vi "Blob ReadEdvr.vi"(8 "error in (no error)":errorcluster, 11 "Blob in":refnum<class "Blob.lvclass">) -> (0 "error out":errorcluster, 2 "Edvr":T1, 3 "Blob out":refnum<class "Blob.lvclass">)   [LabVIEW 2020, in "OpenLvVision_OpenCv.lvlib" / "Blob.lvclass"]
uses:
  Blob.lvclass
  _LvHelpers/EdvrObject/EdvrObject.lvclass
  C:/Users/lukas/Downloads/OpenLvVision_OpenCv/SourceCode/LabView/OpenLvVision_OpenCv/_LvHelpers/EdvrObject/EdvrObject.lvclass
  C:/Users/lukas/Downloads/OpenLvVision_OpenCv/SourceCode/LabView/OpenLvVision_OpenCv/DNN/Blob/Blob.lvclass
  _LvHelpers/EdvrObject/TypeDef/Edvr.ctl
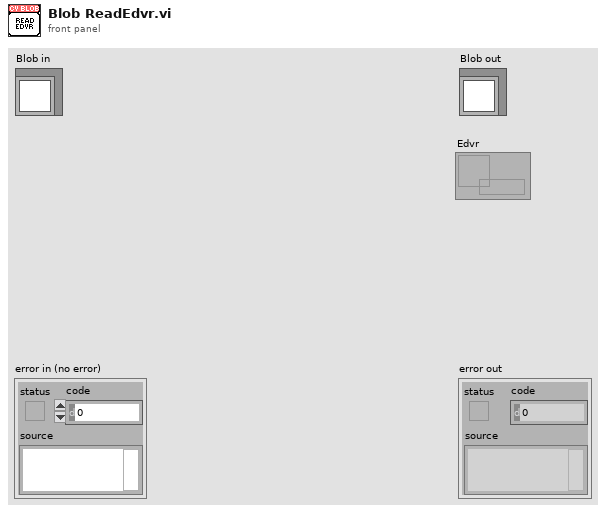
[diagram p1: front panel]
types:
  T1 = typedef "OpenLvVision_OpenCv.lvlib/EdvrObject.lvclass/Edvr.ctl" = refnum<data-value>
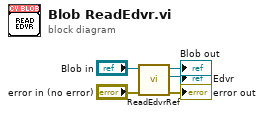
[diagram p0: block diagram]
diagram:
  n1 = call "ReadEdvrRef.vi"("error in (no error)"="error in (no error)", "EdvrObject in"="Blob in") -> ("error out"=→"error out":errorcluster, "Edvr"=→"Edvr":T1, "EdvrObject out"=→"Blob out":refnum<class "Blob.lvclass">)  [unwired: 7 in]
